vi "ProportionalValveTester.vi"() -> ()   [LabVIEW 2019]
uses:
  <vilib>/myRIO/Instrument Drivers/Onboard IO/PWM/typedefs/PWM Reference.ctl
  <vilib>/myRIO/Common/Instrument Driver Framework/Utilities/typedefs/myRIO Generic Hardware Reference.ctl
  <vilib>/myRIO/Common/Instrument Driver Framework/Utilities/typedefs/Hardware Version Enum.ctl
  <vilib>/myRIO/Common/Instrument Driver Framework/Utilities/typedefs/myRIO v1.0 Reference.ctl
  <vilib>/myRIO/Common/Instrument Driver Framework/Utilities/typedefs/Generic FPGA Reference.ctl
  <vilib>/myRIO/Common/Instrument Driver Framework/myRIO v1.0/PWM/typedefs/PWM Channels Enum.ctl
  <vilib>/myRIO/Instrument Drivers/Onboard IO/PWM/typedefs/PWM Configuration.ctl
  <vilib>/userDefined/High Color/nirio_resource_hc.ctl
  <vilib>/myRIO/Instrument Drivers/Onboard IO/AI/typedefs/AI Reference.ctl
  <vilib>/myRIO/Common/Instrument Driver Framework/myRIO v1.0/AI/typedefs/AI Channels List.ctl
  <vilib>/myRIO/Common/Instrument Driver Framework/myRIO v1.0/AI/typedefs/AI Channels Enum.ctl
  <vilib>/myRIO/Common/Instrument Driver Framework/Utilities/typedefs/Analog Scaling Constants List.ctl
  <vilib>/myRIO/Common/Instrument Driver Framework/Utilities/typedefs/Analog Scaling Constants.ctl
  <vilib>/myRIO/Common/Instrument Driver Framework/Utilities/vis/Is FPGA Ref Available.vi
  <vilib>/myRIO/Common/Instrument Driver Framework/myRIO v1.0/AI/vis/myRIO v1.1 Open AI.vi
  <vilib>/myRIO/Instrument Drivers/Onboard IO/AI/vis/Read.vi
  <vilib>/myRIO/Common/Instrument Driver Framework/myRIO v1.0/PWM/vis/myRIO v1.1 Open PWM.vi
  <vilib>/myRIO/Instrument Drivers/Onboard IO/PWM/vis/Set Duty Cycle and Frequency.vi
  <vilib>/myRIO/Common/Instrument Driver Framework/Utilities/vis/Validate Channels.vi
  <vilib>/myRIO/Common/Instrument Driver Framework/myRIO v1.0/AI/vis/myRIO v1.0 Reserve AI.vi
  <vilib>/myRIO/Common/Instrument Driver Framework/myRIO v1.0/PWM/vis/myRIO v1.0 Reserve PWM.vi
  <vilib>/myRIO/Common/Instrument Driver Framework/myRIO v1.0/UART/vis/myRIO v1.0 Close UART.vi
  <vilib>/myRIO/Common/Instrument Driver Framework/myRIO v1.0/AI/vis/myRIO v1.0 Build MUX Configuration AI.vi
  <vilib>/myRIO/Common/Instrument Driver Framework/myRIO v1.0/Resource Manager/vis/myRIO v1.0 Reserve Channel List.vi
  <vilib>/myRIO/Common/Instrument Driver Framework/myRIO v1.0/PWM/vis/myRIO v1.0 Build MUX Configuration PWM.vi
  <vilib>/myRIO/Common/Instrument Driver Framework/myRIO v1.0/Resource Manager/vis/myRIO v1.0 Reserve Channel.vi
  <vilib>/myRIO/Common/Instrument Driver Framework/myRIO v1.0/Resource Manager/vis/myRIO v1.0 Unreserve Channel.vi
  <vilib>/myRIO/Common/Instrument Driver Framework/myRIO v1.0/Resource Manager/vis/myRIO v1.0 Create Configuration List.vi
  <vilib>/myRIO/Common/Instrument Driver Framework/myRIO v1.0/Resource Manager/vis/myRIO v1.0 Build Mutex Name.vi
  <vilib>/Utility/VariantDataType/GetNumericInfo.vi
  <vilib>/Utility/error.llb/Error Cluster From Error Code.vi
  <vilib>/myRIO/Common/Instrument Driver Framework/myRIO v1.0/myRIO v1.1 Open.vi
  <vilib>/myRIO/Common/Instrument Driver Framework/Utilities/vis/IO Manager.vi
  <vilib>/myRIO/Common/Instrument Driver Framework/Utilities/vis/Configuration Manager.vi
  <vilib>/myRIO/Common/Instrument Driver Framework/myRIO v1.0/Resource Manager/vis/myRIO v1.0 Configure IO.vi
  <vilib>/myRIO/Common/Instrument Driver Framework/myRIO v1.0/myRIO v1.0 Close.vi
  <vilib>/myRIO/Common/Instrument Driver Framework/myRIO v1.0/PWM/vis/myRIO v1.0 Write PWM.vi
  <vilib>/myRIO/Common/Instrument Driver Framework/myRIO v1.0/AI/vis/myRIO v1.0 Get Scaling Constants AI.vi
  <vilib>/myRIO/Common/Instrument Driver Framework/myRIO v1.0/AI/vis/myRIO v1.0 Read AI.vi
  <vilib>/imath/engines/lvmath2/RunTimeEngine/Managers/WorkSpace/UID Generator.vi
  <vilib>/imath/engines/lvmath2/RunTimeEngine/RunTimeType/NIMS_RunTimeType_From StrictType (excl LVString).vi
  <instcachedir>/0/NIMS_RunTimeType_From StrictType (excl LVString)_D8AFBA86A94845AAA577C895450664BD.lvgen/NIMS_RunTimeType_From StrictType (excl LVString)_D8AFBA86A94845AAA577C895450664BD_000.vi
  <vilib>/imath/engines/lvmath2/RunTimeEngine/LocalVariableDefStatement/MC_LocalVariableDefStatement_Display.vi
  <vilib>/imath/engines/lvmath2/RunTimeEngine/Managers/SymbolTable/Clear UID.vi
  <vilib>/imath/engines/lvmath2/RunTimeEngine/NodeEndStatement/NIMS_NodeEndStatement_Output.vi
  <instcachedir>/0/NIMS_NodeEndStatement_Output_53EC0D466D134D7ABD903AC30B43404B.lvgen/NIMS_NodeEndStatement_Output_53EC0D466D134D7ABD903AC30B43404B_001.vi
  <vilib>/imath/engines/lvmath2/RunTimeEngine/ErrorHandling/NIMS_Finalize Error.vi
  <vilib>/addons/control/pid/pid.llb/PID (DBL).vi
  <vilib>/myRIO/Common/Instrument Driver Framework/Utilities/vis/FPGA Ref Manager.vi
  <vilib>/myRIO/Common/Instrument Driver Framework/myRIO v1.0/myRIO v1.0 Reset FPGA.vi
  <vilib>/myRIO/Common/Instrument Driver Framework/myRIO v1.0/IRQ/vis/myRIO v1.0 IRQ Info FGV.vi
  <vilib>/myRIO/Common/Instrument Driver Framework/myRIO v1.0/IRQ/vis/myRIO v1.0 Timer IRQ Info FGV.vi
  <vilib>/myRIO/Common/Instrument Driver Framework/myRIO v1.0/IRQ/vis/myRIO v1.0 ISR Agent.vi
  <vilib>/myRIO/Instrument Drivers/Utilities/vis/Reset Index.vi
  <vilib>/myRIO/Common/Instrument Driver Framework/myRIO v1.0/Resource Manager/vis/myRIO v1.0 Block Write Resource Manager.vi
  <vilib>/myRIO/Express VI/Onboard IO/PWM/PWM Express VI.xnode
  <vilib>/myRIO/Instrument Drivers/Onboard IO/PWM/vis/myRIO PWM Open.xnode
  <vilib>/myRIO/Express VI/Onboard IO/AI/AI Express VI.xnode
  <vilib>/myRIO/Instrument Drivers/Onboard IO/AI/vis/myRIO AI Open.xnode
  <vilib>/myRIO/Instrument Drivers/Onboard IO/PWM/PWM.lvlib
  <vilib>/myRIO/Instrument Drivers/Onboard IO/AI/AI.lvlib
  <vilib>/imath/engines/lvmath2/RunTimeEngine/Managers/SymbolTable/NIMS_WorkSpace.lvlib
  <vilib>/addons/control/pid/NI_PID_pid.lvlib
  <vilib>/ptbypt/NI_PtbyPt.lvlib
  <vilib>/myRIO/Instrument Drivers/Utilities/Utilities.lvlib
panel:
  in  "Setpoint Duty":dbl(slide) scale=0.0..1.0
  in  "s":bool
  out "Triangle":dbl format="%#.3g"
  in  "stop":bool
  out "VA_sensor":dbl format="%#.3g"
  out "Pressures Receiver":cluster{dbl, dbl}(knob)={0.0, 8.870406975580165} scale=0.0..120.0
  in  "Setpoint Preceiver":dbl(slide) scale=0.0..100.0
  out "V_Rsensor":dbl format="%#.3g"
  in  "PID Motor":T1={"proportional gain (Kc)"=0.01, "integral time (Ti, min)"=0.005, "derivative time (Td, min)"=0.0} {"derivative time (Td, min)" format="%.3f"; "integral time (Ti, min)" format="%.3f"; "proportional gain (Kc)" format="%.3f"}
  out "Duty cycle Motor":dbl(knob) scale=0.0..1.0
  out "Pressures Actuator":dynamicdata(graph)
  in  "milliseconds to wait":u32=100
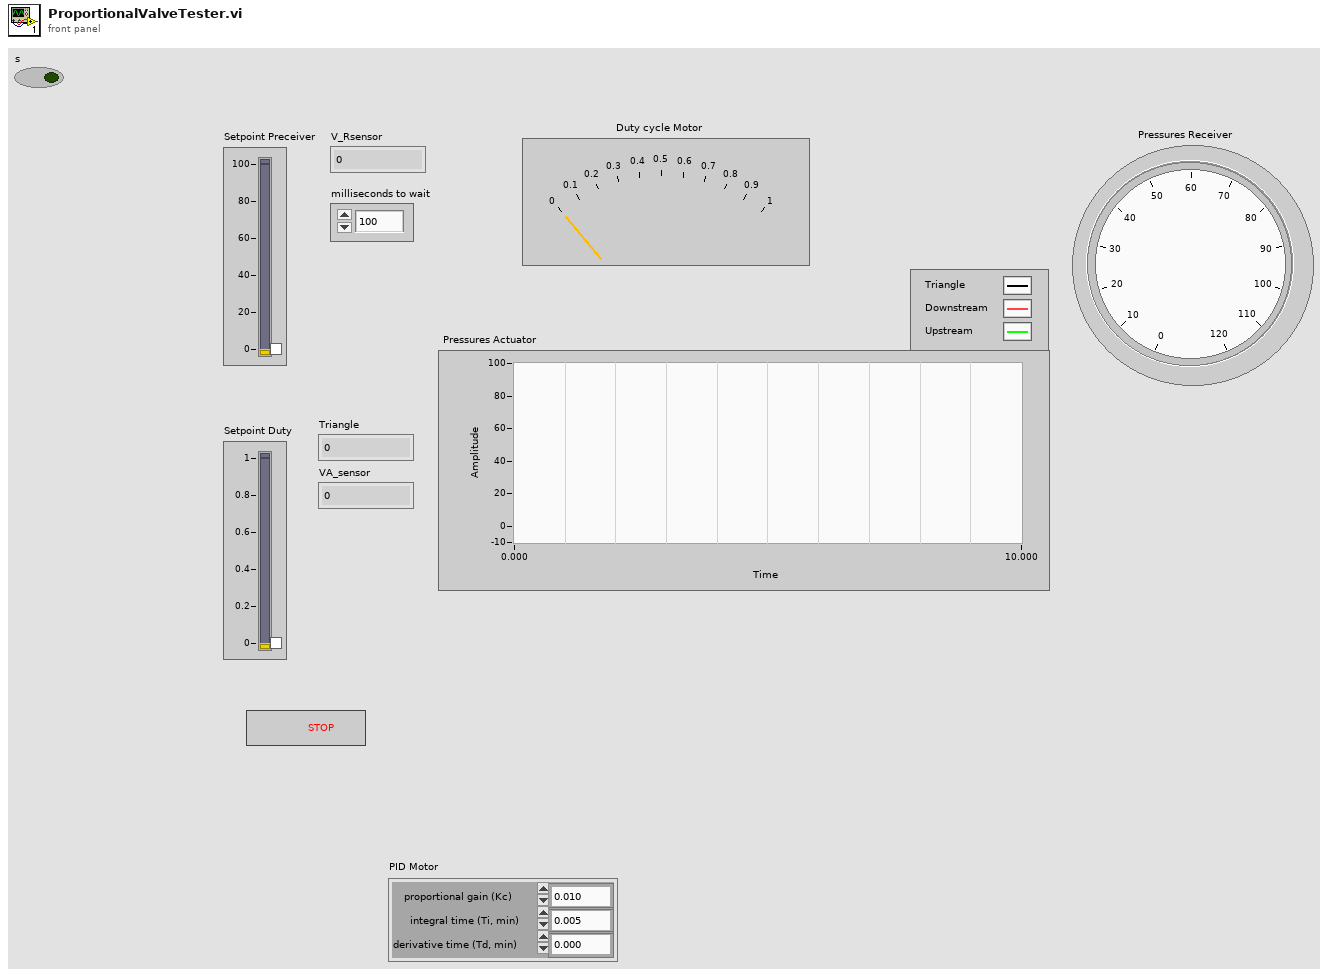
[diagram p1: front panel]
types:
  T1 = cluster{"proportional gain (Kc)":dbl, "integral time (Ti, min)":dbl, "derivative time (Td, min)":dbl}
  T2 = typedef "AI.lvlib/AI Reference.ctl" = cluster{"myRIO Reference":T3, "AI Channels List":T7, "AI Scaling Constants List":T9}
  T3 = typedef "myRIO Generic Hardware Reference.ctl" = cluster{"myRIO Model":T4, "myRIO Hardware Reference":T5}
  T4 = typedef "Hardware Version Enum.ctl" = enum16{"Unknown", "myRIO-1900", "myRIO-1950", "roboRIO", "NI ELVIS RIO CM", "ELVIS III"}
  T5 = typedef "myRIO v1.0 Reference.ctl" = cluster{"Generic FPGA Reference":T6, "Allow multiple opens":bool}
  T6 = typedef "Generic FPGA Reference.ctl" = refnum<k20>
  T7 = typedef "AI Channels List.ctl" = T8[]
  T8 = typedef "AI Channels Enum.ctl" = enum16{"Not Connected", "AudioIn/Left", "AudioIn/Right", "C/AI0", "C/AI1", "A/AI0", "A/AI1", "A/AI2", "A/AI3", "A/AI4", "A/AI5", "A/AI6", "A/AI7", "B/AI0", "B/AI1", "B/AI2", "B/AI3", "B/AI4", "B/AI5", "B/AI6", "B/AI7", "AI/AI0", "AI/AI1", "AI/AI2", "AI/AI3", "A/AI0 (DIFF)", "A/AI1 (DIFF)", "A/AI2 (DIFF)", "A/AI3 (DIFF)", "B/AI0 (DIFF)", "B/AI1 (DIFF)", "B/AI2 (DIFF)", "B/AI3 (DIFF)"}
  T9 = typedef "Analog Scaling Constants List.ctl" = T10[]
  T10 = typedef "Analog Scaling Constants.ctl" = cluster{"LSB Weight (Volts)":dbl, "Offset (Volts)":dbl, "Signed?":bool}
  T11 = typedef "nirio_resource_hc.ctl" = tag
  T12 = typedef "PWM.lvlib/PWM Reference.ctl" = cluster{"myRIO Reference":T3, "PWM Channels Enum":T13, "PWM Configuration":T14}
  T13 = typedef "PWM Channels Enum.ctl" = enum16{"Not Connected", "C/PWM0", "C/PWM1", "A/PWM0", "A/PWM1", "A/PWM2", "A/PWM3", "A/PWM4", "A/PWM5", "A/PWM6", "A/PWM7", "A/PWM8", "A/PWM9", "A/PWM10", "A/PWM11", "A/PWM12", "A/PWM13", "A/PWM14", "A/PWM15", "A/PWM16", "A/PWM17", "A/PWM18", "A/PWM19", "B/PWM0", "B/PWM1", "B/PWM2", "B/PWM3", "B/PWM4", "B/PWM5", "B/PWM6", "B/PWM7", "B/PWM8", "B/PWM9", "B/PWM10", "B/PWM11", "B/PWM12", "B/PWM13", "B/PWM14", "B/PWM15", "B/PWM16", "B/PWM17", "B/PWM18", "B/PWM19", "PWM/PWM0", "PWM/PWM1", "PWM/PWM2", "PWM/PWM3", "PWM/PWM4", "PWM/PWM5", "PWM/PWM6", "PWM/PWM7", "PWM/PWM8", "PWM/PWM9"}
  T14 = typedef "PWM.lvlib/PWM Configuration.ctl" = cluster{"Frequency":dbl, "Duty Cycle":dbl}
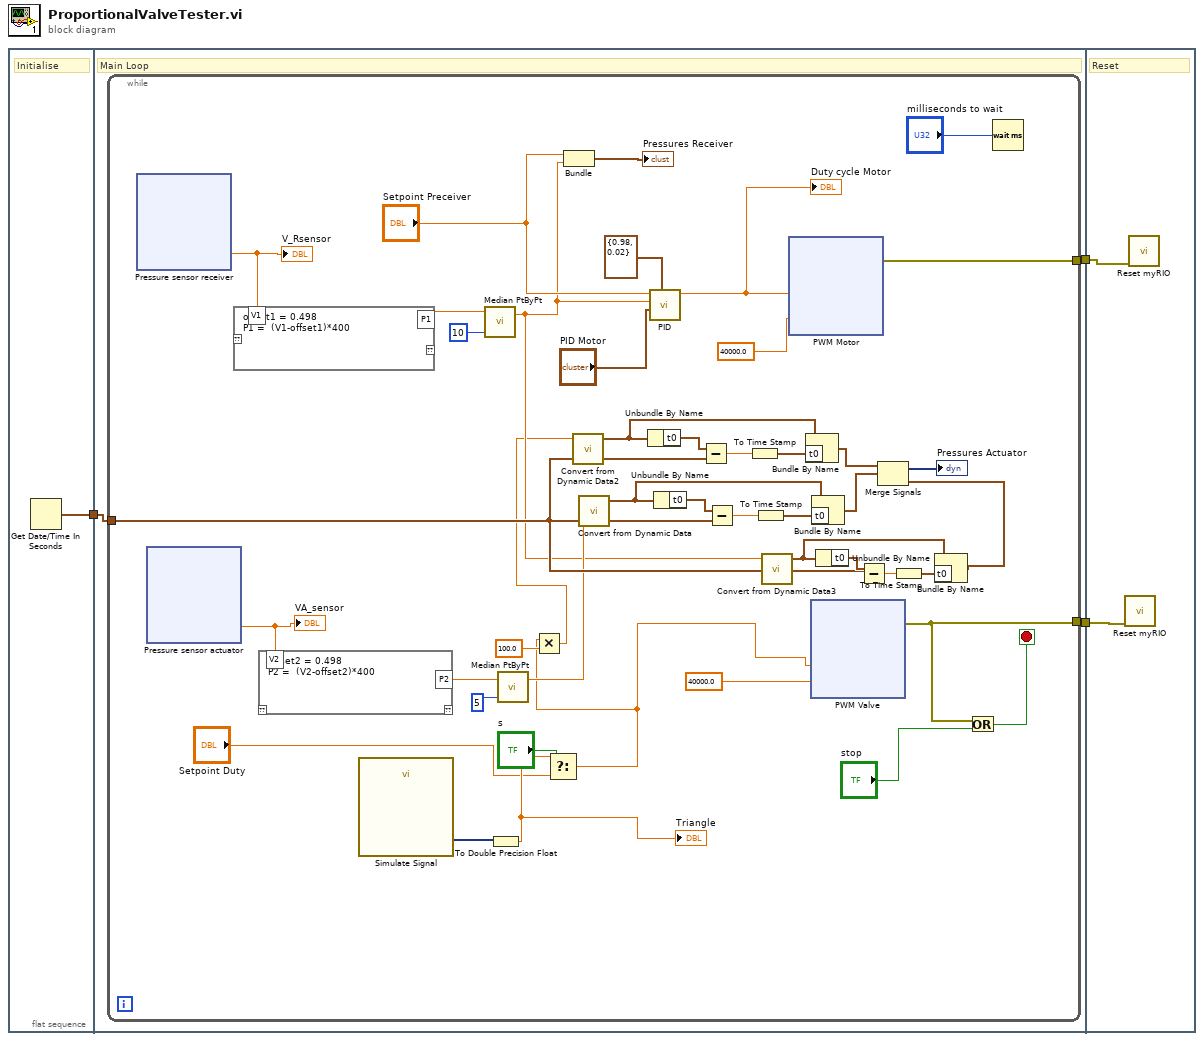
[diagram p0: block diagram]
diagram:
  n1 = flat-sequence {
    tunnel: [w4] -> w3
    tunnel: [w7] -> w2
    tunnel: [w6] -> w1
    tunnel: w3 -> [w5]
    tunnel: w2 -> [w299]
    tunnel: w1 -> [w298]
    frame #0 {
      # "Initialise"
      n2 = Get Date/Time In Seconds() -> (seconds since 1Jan1904=w4:timestamp)
    }
    frame #1 {
      # "Main Loop"
      n3 = while {
        tunnel: [w50] -> w7
        tunnel: [w39] -> w6
        tunnel: w5 -> [w22]
        stop <- w49 stop-if-true
        n4 = xnode "Pressure sensor receiver"() -> ("B/AI0 (Pin 3)"=w19:dbl)  [unwired: 1 in, 1 out]
        "V_Rsensor" <- w19
        n5 = xnode "Pressure sensor actuator"() -> ("B/AI1 (Pin 5)"=w18:dbl)  [unwired: 1 in, 1 out]
        "VA_sensor" <- w18
        n6 = mathscript code="offset1 = 0.498\nP1 =  (V1-offset1)*400"("V1"=w19) -> ("P1"=w41:dbl)  [unwired: 1 in, 1 out]
        n7 = mathscript code="offset2 = 0.498\nP2 =  (V2-offset2)*400"("V2"=w18) -> ("P2"=w48:dbl)  [unwired: 1 in, 1 out]
        n8 = call "Simulate Signal"() -> ("Triangle"=w17:dynamicdata)  [unwired: 14 in, 1 out]
        n9 = call <vilib>:"Median PtByPt.vi"("sample length"=10, "x"=w41) -> ("median"=w14:dbl)  [unwired: 2 in, 1 out]
        n10 = To Double Precision Float(number=w17) -> (double precision float=w9:dbl)
        "Triangle" <- w9
        n11 = call <vilib>:"Median PtByPt.vi"("sample length"=5, "x"=w48) -> ("median"=w20:dbl)  [unwired: 2 in, 1 out]
        n12 = Select(t=w9, s="s", f="Setpoint Duty") -> (s? t:f=w11:dbl)
        n13 = Multiply(x=w11, y=100.0) -> (x*y=w13:dbl)
        n14 = Bundle("Setpoint Preceiver"="Setpoint Preceiver", "median"=w14) -> (→"Pressures Receiver":cluster{"Setpoint Preceiver":dbl, "median":dbl})  [unwired: 1 in]
        n15 = call "Convert from Dynamic Data2"("Dynamic Data Type"=w13) -> ("Waveform"=w32:waveform(dbl))  [unwired: 3 in]
        n16 = call "Convert from Dynamic Data"("Dynamic Data Type"=w20) -> ("Waveform"=w38:waveform(dbl))  [unwired: 3 in]
        n17 = Unbundle By Name(w32) -> ("t0"=w29:timestamp)
        n18 = call-poly <vilib>:"PID.vi"("output range"=cluster{"output high":dbl, "output low":dbl} {"output high"=0.98, "output low"=0.02} ("output range motor"), "PID gains"="PID Motor", "process variable"=w14, "setpoint"="Setpoint Preceiver") -> ("output"=w16:dbl)  [unwired: 6 in, 1 out]
        "Duty cycle Motor" <- w16
        n19 = Unbundle By Name(w38) -> ("t0"=w33:timestamp)
        n20 = Subtract(x=w29, y=w22) -> (x-y=w31:dbl)
        n21 = Subtract(x=w33, y=w22) -> (x-y=w37:dbl)
        n22 = To Time Stamp(1:w31) -> (0:w30:timestamp)
        n23 = To Time Stamp(1:w37) -> (0:w36:timestamp)
        n24 = call "Convert from Dynamic Data3"("Dynamic Data Type"=w14) -> ("Waveform"=w26:waveform(dbl))  [unwired: 3 in]
        n25 = xnode "PWM Motor"("Duty Cycle"=w16, "Frequency [Hz]"=40000.0) -> ("error out"=w39:errorcluster)  [unwired: 1 in]
        n26 = Bundle By Name(cluster=w32, "t0"=w30) -> (w28:waveform(dbl))
        n27 = xnode "PWM Valve"("Duty Cycle"=w11, "Frequency [Hz]"=40000.0) -> ("error out"=w50:errorcluster)  [unwired: 1 in]
        n28 = Bundle By Name(cluster=w38, "t0"=w36) -> (w34:waveform(dbl))
        n29 = Unbundle By Name(w26) -> ("t0"=w23:timestamp)
        n30 = Subtract(x=w23, y=w22) -> (x-y=w25:dbl)
        n31 = To Time Stamp(1:w25) -> (0:w24:timestamp)
        n32 = Bundle By Name(cluster=w26, "t0"=w24) -> (w15:waveform(dbl))
        n33 = Merge Signals(w28, w34, w15) -> (→"Pressures Actuator":dynamicdata)
        n34 = Or(x=w50, y="stop") -> (x .or. y?=w49:bool)
        n35 = Wait (ms)(milliseconds to wait="milliseconds to wait") -> ()  [unwired: 1 out]
      }
    }
    frame #2 {
      # "Reset"
      n36 = call <vilib>:"Reset myRIO.vi"("error in (no error)"=w299) -> ()  [unwired: 10 in, 1 out]
      n37 = call <vilib>:"Reset myRIO.vi"("error in (no error)"=w298) -> ()  [unwired: 10 in, 1 out]
    }
  }
